vi "GetText.vi"(8 "error in":errorcluster, 11 "Engine in":refnum<class "CVT Engine Editor.lvclass">) -> (0 "error out":errorcluster, 1 "additional text":string, 2 "text":string, 3 "Engine out":refnum<class "CVT Engine Editor.lvclass">, 4 "glyph":string)   [LabVIEW 2013, in "CVT Engine Editor.lvclass"]
uses:
  CVT Engine Editor.lvclass
  <vilib>/NI/Tag Bus Data Framework/Configuration Editor/subVIs/Glyphs Status.ctl
  <vilib>/NI/Tag Bus Data Framework/Configuration Editor/Classes/Engine Parent/Engine Parent Editor Node.lvclass
  <vilib>/NI/Tag Bus Data Framework/Configuration Editor/PL Framework Configuration Tool.lvlib
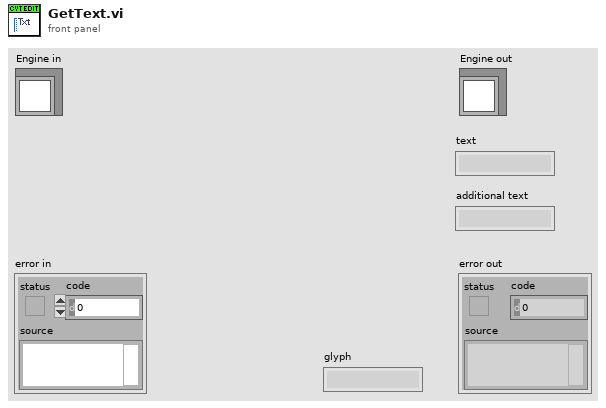
[diagram p1: front panel]
types:
  T1 = typedef "PL Framework Configuration Tool.lvlib/Glyphs Status.ctl" = enum16{"Normal", "Error"}
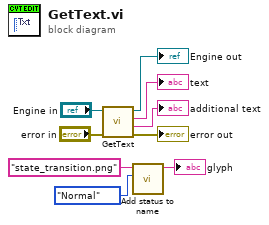
[diagram p0: block diagram]
diagram:
  n1 = call-parent "GetText.vi"("error in"="error in", "Engine in"="Engine in") -> ("error out"=→"error out":errorcluster, "additional text"=→"additional text":string, "text"=→"text":string, "Engine out"=→"Engine out":refnum<class "CVT Engine Editor.lvclass">)  [unwired: 5 in, 1 out]
  n2 = call <vilib>:"Add status to name.vi"("Status"=Glyphs_Status."Normal", "Name"="state_transition.png") -> ("Name with status"=→"glyph":string)  [unwired: 9 in]
